vi "as INT64.vi"(11 "bytes":u8[](array[numeric]) format="%b") -> (3 "INT64":i64)   [LabVIEW 2020, in "MessagePack.lvlib" / "MessagePackNumeric.lvclass"]
uses:
  MessagePackNumeric.lvclass
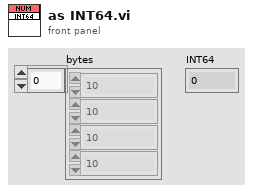
[diagram p1: front panel]
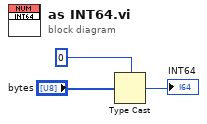
[diagram p0: block diagram]
diagram:
  n1 = Type Cast(type=i64 0 ("INT8"), x="bytes") -> (*(type *) &x=→"INT64":i64)
